vi "CAlex_Param_GV.vi"() -> ()   [LabVIEW 2016]
uses:
  Remote VIs/Configs/CMSMismatch.ctl
panel:
  out "CMSMismatch":T1
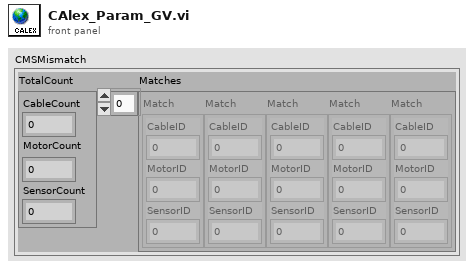
[diagram p1: front panel]
types:
  T1 = typedef "CMSMismatch.ctl" = cluster{"TotalCount":cluster{"CableCount":i32, "MotorCount":i32, "SensorCount":i32}, "Matches":cluster{"CableID":i32, "MotorID":i32, "SensorID":i32}[]}
diagram:
